vi "GetChannels.vi"(8 "error in (no error)":errorcluster, 11 "IviFgen in":refnum<class "IviFgen.lvclass">) -> (0 "error out":errorcluster, 2 "Channels":cluster{"Count":u16, "Channel":T1[]}, 3 "IviFgen out":refnum<class "IviFgen.lvclass">)   [LabVIEW 2018, in "FgenPlugins.lvlib" / "IviFgen.lvclass"]
uses:
  IviFgen.lvclass
  X:/Projects/NistPluggableModules/dev/NistPluggableModules/FGen/FgenPlugins/FgenPluginBaseClass/FgenPluginsBase.lvclass
  TypeDefs/Channel.ctl
  FgenPluginBaseClass/FgenPluginsBase.lvclass/FgenPluginsBase.ctl
  FgenPluginBaseClass/Accessors/Read Channels.vi
  FgenPluginBaseClass/FgenPluginsBase.lvclass
  FgenPlugins.lvlib
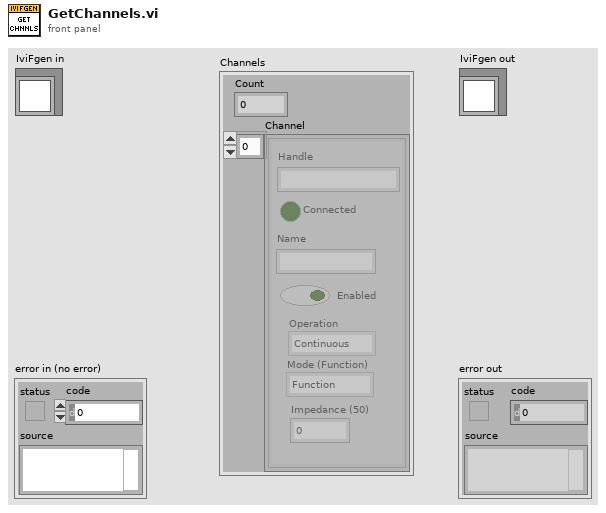
[diagram p1: front panel]
types:
  T1 = typedef "FgenPlugins.lvlib/Channel.ctl" = cluster{"Name":string, "Enabled":bool, "Operation":enum16{"Continuous", "Burst"}, "Impedance (50)":dbl, "Handle":string, "Connected":bool, "Mode (Function)":enum16{"Function", "Arbitrary", "Sequence"}}
  T2 = typedef "Channel.ctl" = cluster{"Name":string, "Enabled":bool, "Operation":enum16{"Continuous", "Burst"}, "Impedance (50)":dbl, "Handle":string, "Connected":bool, "Mode (Function)":enum16{"Function", "Arbitrary", "Sequence"}}
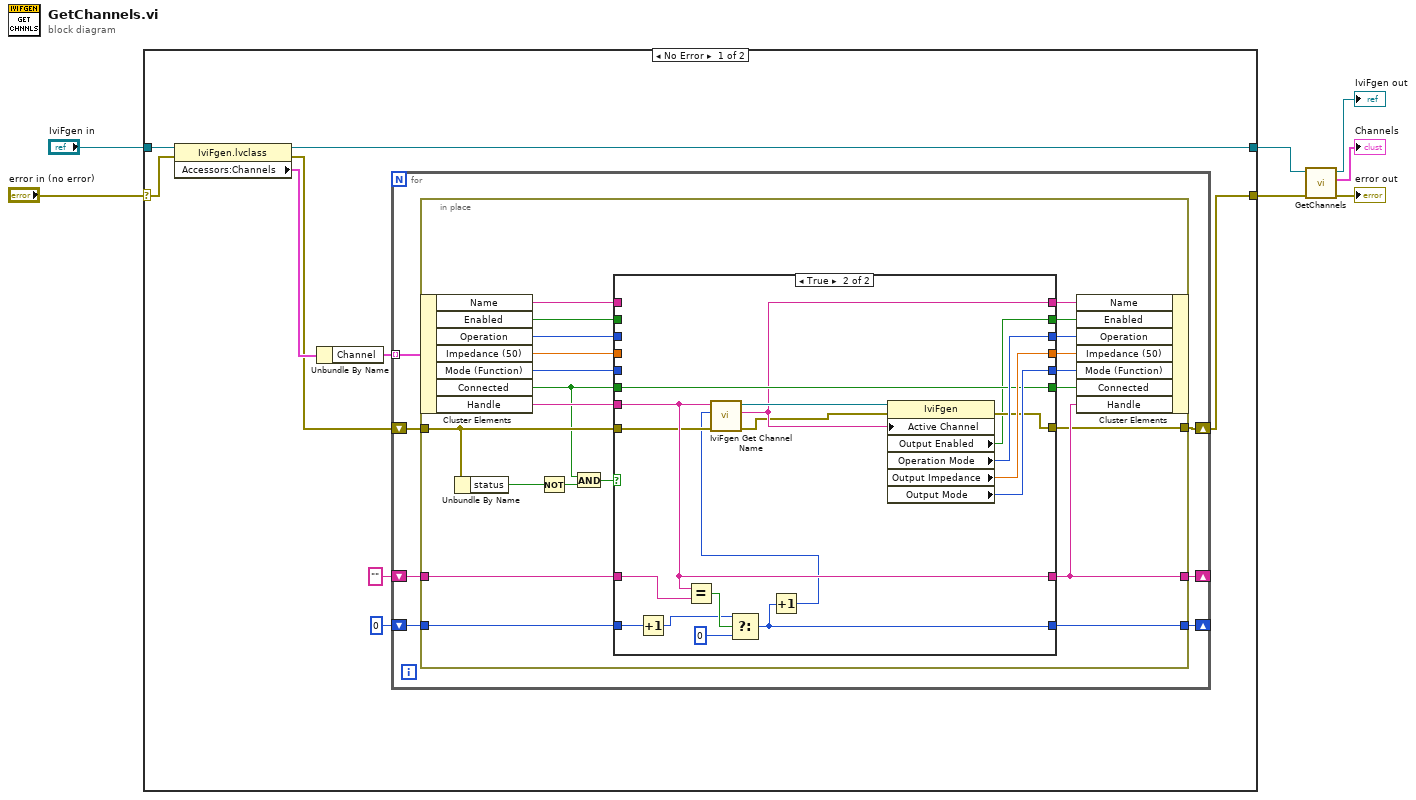
[diagram p0: block diagram]
diagram:
  n1 = case shown="No Error" "error in (no error)" {
    selector: "error in (no error)" -> [w14 w73]
    tunnel: "IviFgen in" -> [w16 w74]
    tunnel: [w15 w74] -> w3
    tunnel: [w8 w73] -> w1
    frame No Error {
      n2 = property class="IviFgen.lvclass"(reference=w16, error in=w14) -> (reference out=w15:refnum<class "IviFgen.lvclass">, error out=w9:errorcluster, "Accessors:Channels"=w13:cluster{"Count":u16, "Channel":T2[]})
      n3 = Unbundle By Name(w13) -> ("Channel"=w12:T2[])
      n4 = for {
        tunnel: w12 -> [w23] mode=indexing
        shift-right: [w22] -> _
        shift-left: "" ("Handle") -> [w21]
        shift-right: [w20] -> _
        shift-left: 0 -> [w19]
        shift-right: [w17] -> w8
        shift-left: w9 -> [w18]
        n5 = in-place {
          in-place-border: [w30] -> w22
          in-place-border: w21 -> [w45]
          in-place-border: [w44] -> w20
          in-place-border: w19 -> [w43]
          in-place-border: w18 -> [w28]
          in-place-border: [w29] -> w17
          n6 = in-place-cluster #1(w23) -> ("Name"=w35:string, "Enabled"=w34:bool, "Operation"=w33:enum16{"Continuous", "Burst"}, "Impedance (50)"=w32:dbl, "Mode (Function)"=w31:enum16{"Function", "Arbitrary", "Sequence"}, "Connected"=w24:bool, "Handle"=w36:string)
          n7 = Unbundle By Name(w28) -> ("status"=w26:bool)
          n8 = Not(x=w26) -> (.not. x?=w27:bool)
          n9 = And(x=w24, y=w27) -> (x .and. y?=w25:bool)
          n10 = case shown="True" w25 {
            tunnel: w36 -> [w49 w72]
            tunnel: [w49 w72] -> w30
            tunnel: w45 -> [_ w71]
            tunnel: [w48 w60] -> w44
            tunnel: w43 -> [w48 w68]
            tunnel: w28 -> [w47 w66]
            tunnel: [w54 w56] -> w42
            tunnel: [w53 w58] -> w41
            tunnel: [w52 w65] -> w40
            tunnel: [w51 w64] -> w37
            tunnel: [w50 w63] -> w39
            tunnel: [w46 w61] -> w38
            tunnel: w35 -> [w54 _]
            tunnel: w34 -> [w53 _]
            tunnel: w33 -> [w52 _]
            tunnel: w32 -> [w51 _]
            tunnel: w31 -> [w50 _]
            tunnel: [w47 w62] -> w29
            tunnel: w24 -> [w46 w61]
            frame False {
            }
            frame True {
              n11 = Increment(x=w68) -> (x+1=w67:i32)
              n12 = Equal?(x=w72, y=w71) -> (x = y?=w70:bool)
              n13 = Select(t=w67, s=w70, f=0) -> (s? t:f=w60:i32)
              n14 = Increment(x=w60) -> (x+1=w59:i32)
              n15 = call <vilib>:"IviFgen Get Channel Name.vi"("error in (no error)"=w66, "Channel Index (1)"=w59, "instrument handle"=w72) -> ("error out"=w55:errorcluster, "Channel Name"=w56:string, "instrument handle out"=w57:refnum<k15>)  [unwired: 6 in]
              n16 = property class="IviFgen"(reference=w57, error in=w55, "Active Channel"=w56) -> (error out=w62:errorcluster, "Output Enabled"=w58:bool, "Operation Mode"=w65:i32, "Output Impedance"=w64:dbl, "Output Mode"=w63:i32)  [unwired: 1 out]
            }
          }
          n17 = in-place-cluster #1("Name"=w42, "Enabled"=w41, "Operation"=w40, "Impedance (50)"=w37, "Mode (Function)"=w39, "Connected"=w38, "Handle"=w30) -> ()  [unwired: 1 out]
        }
      }
    }
    frame Error {
    }
  }
  n18 = call-parent "GetChannels.vi"("error in (no error)"=w1, "FgenPluginsBase in"=w3) -> ("error out"=→"error out":errorcluster, "Channels"=→"Channels":cluster{"Count":u16, "Channel":T1[]}, "FgenPluginsBase out"=→"IviFgen out":refnum<class "IviFgen.lvclass">)  [unwired: 7 in]
